vi "Run Post-Render Delimiter.vi"(8 "Error In":errorcluster, 10 "Output In":string, 11 "Context In":refnum<class "Context.lvclass">) -> (0 "Error Out":errorcluster, 2 "Output Out":string, 3 "Context Out":refnum<class "Context.lvclass">)   [LabVIEW 2018, in "Toolkit.lvlib" / "Context.lvclass"]
uses:
  Context.lvclass
  Context.lvclass/Context.ctl
  Hooks/Render/Delimiter/Delimiter.lvclass
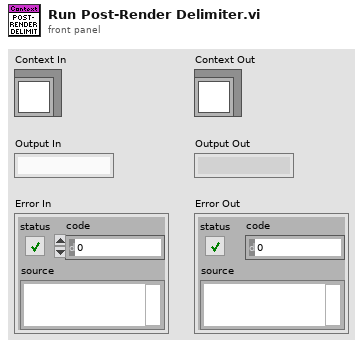
[diagram p1: front panel]
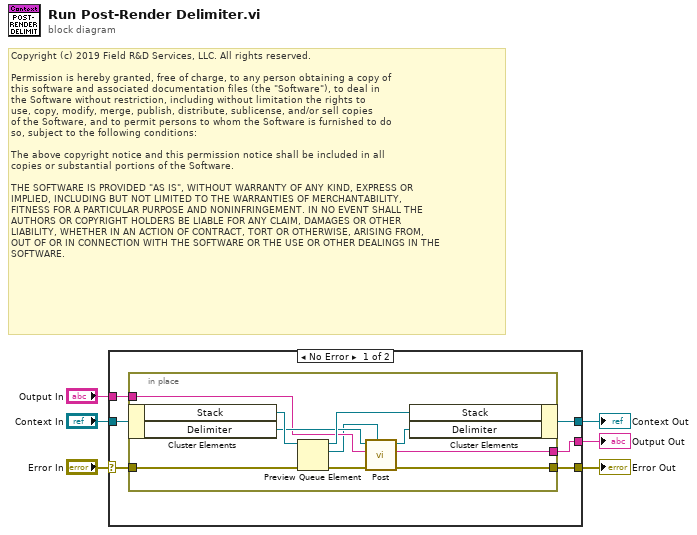
[diagram p0: block diagram]
diagram:
  # "Copyright (c) 2019 Field R&D Services, LLC. All rights reserved.\n\nPermission is hereby granted, free of charge, to any person obtaining a copy of\nthis software and associated documentation files (the \"Software\"), to deal in\nthe Software without restriction, including without limitation the rights to\nuse, copy, modify, merge, publish, distribute, sublicense, and/or sell copies\nof the Software, and to permit persons to whom the Software is furnished to do\nso, subject to the following conditions:\n\nThe above copyright notice and this permission notice shall be included in all\ncopies or substantial portions of the Software.\n\nTHE SOFTWARE IS PROVIDED \"AS IS\", WITHOUT WARRANTY OF ANY KIND, EXPRESS OR\nIMPLIED, INCLUDING BUT NOT LIMITED TO THE WARRANTIES OF MERCHANTABILITY,\nFITNESS FOR A PARTICULAR PURPOSE AND NONINFRINGEMENT. IN NO EVENT SHALL THE\nAUTHORS OR COPYRIGHT HOLDERS BE LIABLE FOR ANY CLAIM, DAMAGES OR OTHER\nLIABILITY, WHETHER IN AN ACTION OF CONTRACT, TORT OR OTHERWISE, ARISING FROM,\nOUT OF OR IN CONNECTION WITH THE SOFTWARE OR THE USE OR OTHER DEALINGS IN THE\nSOFTWARE."
  n1 = case shown="No Error" "Error In" {
    selector: "Error In" -> [w12 w24]
    tunnel: "Context In" -> [w10 w25]
    tunnel: [w11 w25] -> w4
    tunnel: [w8 w24] -> w3
    tunnel: "Output In" -> [w9 w23]
    tunnel: [w7 w23] -> w1
    frame No Error {
      n2 = in-place {
        in-place-border: w12 -> [w20]
        in-place-border: w9 -> [w14]
        in-place-border: [w16] -> w8
        in-place-border: [w15] -> w7
        n3 = in-place-cluster #1(w10) -> ("Stack"=w22:refnum<queue>, "Delimiter"=w18:refnum<class "Delimiter.lvclass">)
        n4 = Preview Queue Element(queue=w22, error in (no error)=w20) -> (queue out=w21:refnum<queue>, element=w13:refnum<class "Datum.lvclass">, error out=w19:errorcluster)  [unwired: 1 in, 1 out]
        n5 = call-dynamic "Post.vi"("Datum"=w13, "Error In"=w19, "Output In"=w14, "Render Delimiter In"=w18) -> ("Error Out"=w16:errorcluster, "Output Out"=w15:string, "Render Delimiter Out"=w17:refnum<class "Delimiter.lvclass">)  [unwired: 5 in]
        n6 = in-place-cluster #1("Stack"=w21, "Delimiter"=w17) -> (w11:refnum<class "Context.lvclass">)
      }
    }
    frame Error {
    }
  }
  "Context Out" <- w4
  "Error Out" <- w3
  "Output Out" <- w1
